vi "Config-Default.vi"() -> (0 "Default Config":T1)   [LabVIEW 2024, in "GLF.lvlib" / "Engine.lvclass"]
uses:
  Engine.lvclass
  Engine.lvclass/Engine.ctl
  Config--cluster.ctl
  VSync--enum.ctl
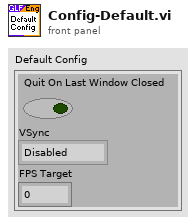
[diagram p1: front panel]
types:
  T1 = typedef "GLF.lvlib/Engine.lvclass/Config--cluster.ctl" = cluster{"Quit On Last Window Closed":bool, "VSync":T2, "FPS Target":dbl}
  T2 = typedef "GLF.lvlib/Engine.lvclass/VSync--enum.ctl" = enum16{"Disabled", "Enabled", "Adaptative"}
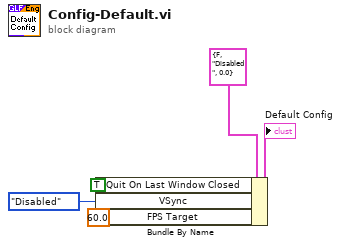
[diagram p0: block diagram]
diagram:
  n1 = Bundle By Name(cluster=T1 {"Quit On Last Window Closed"=FALSE, "VSync"=enum."Disabled", "FPS Target"=0.0} ("Default Config"), "Quit On Last Window Closed"=TRUE ("Close On SDL Quit?"), "VSync"=VSync--enum."Disabled", "FPS Target"=60.0) -> (→"Default Config":T1)
